vi "Check If Double Scanner.vi"(11 "Scanner in":refnum<class "Scanner.lvclass">) -> (2 "Is Double Scanner?":bool)   [LabVIEW 2017, in "Scanner.lvclass"]
uses:
  Scanner.lvclass
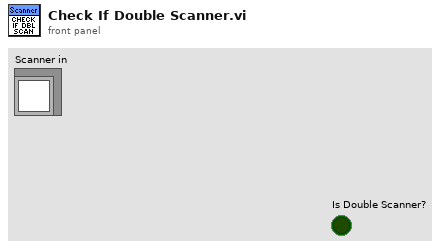
[diagram p1: front panel]
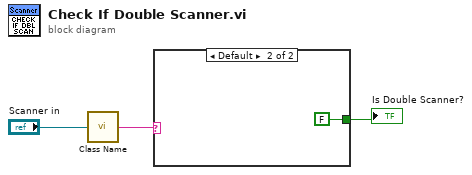
[diagram p0: block diagram]
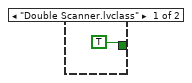
[diagram p2: hidden frame]
diagram:
  n1 = call "Class Name.vi"("LabVIEW Object"="Scanner in") -> ("Classname"=w3:string)
  n2 = case shown="Default" w3 {
    tunnel: [TRUE ("Is Double Scanner?") FALSE ("Is Double Scanner?")] -> w1
    frame "Double Scanner.lvclass" {
    }
    frame Default {
    }
  }
  "Is Double Scanner?" <- w1
